vi "FGV Gaszuordnung Gas-Auswahl.vi"(6 "Aktion":T4, 8 "Graphen":T1, 10 "Auswahlfelder":T2, 11 "aktiver Graph":i32) -> (0 "Graphen":T1, 2 "Auswahlfelder OUT":T2, 3 "aktiver Graph":i32)   [LabVIEW 2020, in "Gaszuordnung AO.lvlib"]
uses:
  Gaszuordnung AO.lvlib
  Auswahlfelder Anzeige.ctl
  Visualisierungs Elemente/Auswahlfeld.ctl
  FGV Gaszuordnung Gas-Auswahl Aktion.ctl
  Grafik/Graphen Auswahl.ctl
  Allgemein/allgemeine Sub-VIs.lvlib
  Grafik/Grafik.lvlib
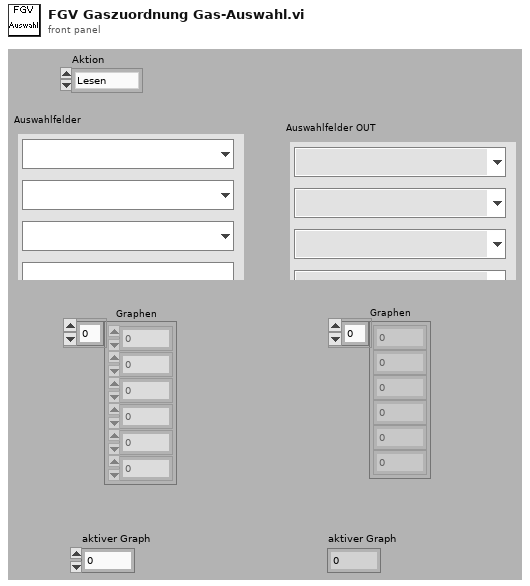
[diagram p1: front panel]
types:
  T1 = typedef "Grafik.lvlib/Graphen Auswahl.ctl" = u16[]
  T2 = typedef "Gaszuordnung AO.lvlib/Auswahlfelder Anzeige.ctl" = cluster{"Auswahl":T3, "Auswahl 2":T3, "Auswahl 3":T3, "Auswahl 4":T3, "Auswahl 5":T3, "Auswahl 6":T3, "Auswahl 7":T3, "Auswahl 8":T3, "Auswahl 9":T3, "Auswahl 10":T3, "Auswahl 11":T3, "Auswahl 12":T3, "Auswahl 13":T3, "Auswahl 14":T3, "Auswahl 15":T3, "Auswahl 16":T3}
  T3 = typedef "Auswahlfeld.ctl" = u16
  T4 = typedef "Gaszuordnung AO.lvlib/FGV Gaszuordnung Gas-Auswahl Aktion.ctl" = enum16{"Lesen", "AO Auswahl", "Graph Auswahl", "aktiver Graph", "laden", "speichern"}
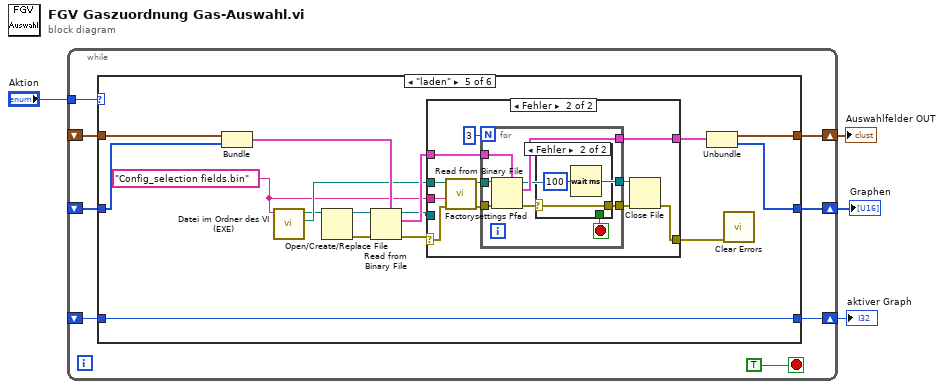
[diagram p0: block diagram]
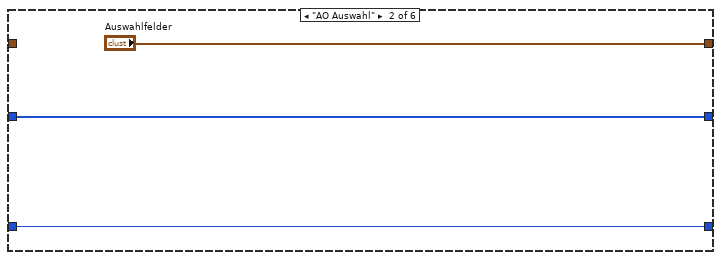
[diagram p3: hidden frame]
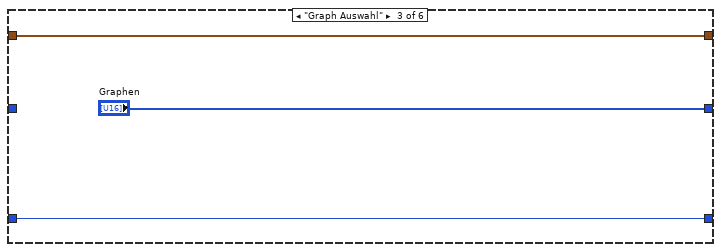
[diagram p4: hidden frame]
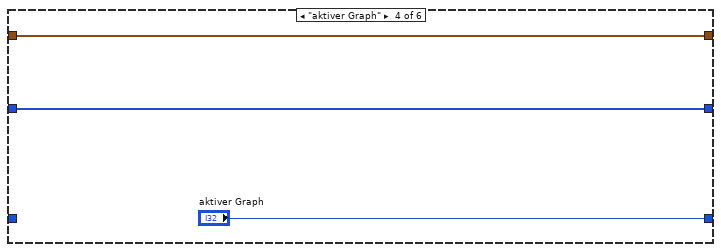
[diagram p5: hidden frame]
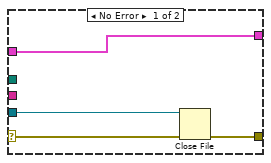
[diagram p6: hidden frame]
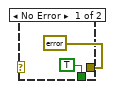
[diagram p7: hidden frame]
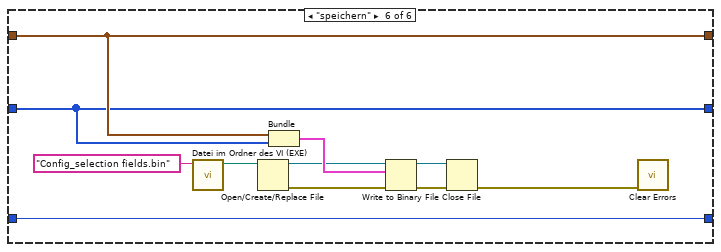
[diagram p8: hidden frame]
diagram:
  n1 = while {
    tunnel: "Aktion" -> [w11]
    shift-right: [w10] -> w3
    shift-left: _ -> [w9]
    shift-right: [w8] -> w2
    shift-left: _ -> [w7]
    shift-right: [w6] -> w1
    shift-left: _ -> [w5]
    stop <- TRUE stop-if-true
    n2 = case shown="\"laden\"" w11 {
      tunnel: [w15 "Auswahlfelder" w20 w22 w37 w77] -> w10
      tunnel: w9 -> [w15 _ w20 w22 w40 w77]
      tunnel: [w14 w17 "Graphen" w23 w36 w76] -> w8
      tunnel: w7 -> [w14 w17 _ w23 w39 w76]
      tunnel: [w13 w16 w19 "aktiver Graph" w35 w74] -> w6
      tunnel: w5 -> [w13 w16 w19 _ w35 w74]
      frame "Lesen", Default {
      }
      frame "AO Auswahl" {
      }
      frame "Graph Auswahl" {
      }
      frame "aktiver Graph" {
      }
      frame "laden" {
        w28 = "Config_selection fields.bin" ("Dateiname")
        n3 = Bundle("Auswahlfelder"=w40, "Graphen"=w39) -> (w38:cluster{"Auswahlfelder":T2, "Graphen":T1})  [unwired: 1 in]
        n4 = call "Datei im Ordner des VI (EXE).vi"("Dateiname"=w28) -> ("Ordner des Haupt-VIs"=w32:path, "Dateipfad im Ordner des Haupt-VIs"=w27:path)  [unwired: 8 in, 1 out]
        n5 = Open/Create/Replace File(file path (use dialog)=w27) -> (refnum out=w26:refnum<file>, error out=w25:errorcluster)  [unwired: 5 in, 1 out]
        n6 = Read from Binary File(5:w38, 8:w25, 11:w26) -> (0:w34:errorcluster, 2:w33:cluster{"Auswahlfelder":T2, "Graphen":T1}, 3:w31:refnum<file>)  [unwired: 3 in, 1 out]
        n7 = case shown="Fehler" w34 {
          selector: w34 -> [w43 w47]
          tunnel: w32 -> [_ w48]
          tunnel: w33 -> [w44 w46]
          tunnel: [w44 w54] -> w29
          tunnel: [w41 w52] -> w30
          tunnel: w31 -> [w42 _]
          tunnel: w28 -> [_ w45]
          frame No Error {
            n8 = Close File(refnum=w42, error in=w43) -> (error out=w41:errorcluster)  [unwired: 1 out]
          }
          frame Error {
            n9 = call "Factorysettings Pfad.vi"("error in (no error)"=w47, "Dateiname"=w45, "Ordner des Haupt-VIs"=w48) -> ("error out"=w49:errorcluster, "Pfad Factorysettings"=w50:path)  [unwired: 7 in]
            n10 = for {
              N: 3 -> [_]
              tunnel: w49 -> [w61]
              tunnel: w50 -> [w60]
              tunnel: [w59] -> w54
              tunnel: [w58] -> w53
              tunnel: [w57] -> w51
              tunnel: w46 -> [w56]
              stop <- w62 stop-if-true
              n11 = Read from Binary File(5:w56, 8:w61, 11:w60) -> (0:w63:errorcluster, 2:w59:cluster{"Auswahlfelder":T2, "Graphen":T1}, 3:w57:refnum<file>)  [unwired: 3 in, 1 out]
              n12 = case shown="Fehler" w63 {
                selector: w63 -> [_ w66]
                tunnel: [TRUE _] -> w62
                tunnel: [errorcluster {"status"=FALSE, "code"=0, "source"=""} ("error IO") w66] -> w58
                frame No Error {
                }
                frame Error {
                  n13 = Wait (ms)(milliseconds to wait=u32 100 ("Zu wartende ms")) -> ()  [unwired: 1 out]
                }
              }
            }
            n14 = Close File(refnum=w51, error in=w53) -> (error out=w52:errorcluster)  [unwired: 1 out]
          }
        }
        n15 = Unbundle(w29) -> ("Auswahlfelder"=w37:T2, "Graphen"=w36:T1)
        n16 = call <vilib>:"Clear Errors.vi"("error in (no error)"=w30) -> ()  [unwired: 5 in, 2 out]
      }
      frame "speichern" {
        n17 = call "Datei im Ordner des VI (EXE).vi"("Dateiname"="Config_selection fields.bin") -> ("Dateipfad im Ordner des Haupt-VIs"=w73:path)  [unwired: 8 in, 2 out]
        n18 = Open/Create/Replace File(file path (use dialog)=w73) -> (refnum out=w72:refnum<file>, error out=w71:errorcluster)  [unwired: 5 in, 1 out]
        n19 = Bundle("Auswahlfelder"=w77, "Graphen"=w76) -> (w75:cluster{"Auswahlfelder":T2, "Graphen":T1})  [unwired: 1 in]
        n20 = Write to Binary File(file (use dialog)=w72, data=w75, error in=w71) -> (refnum out=w68:refnum<file>, error out=w70:errorcluster)  [unwired: 3 in, 1 out]
        n21 = Close File(refnum=w68, error in=w70) -> (error out=w69:errorcluster)  [unwired: 1 out]
        n22 = call <vilib>:"Clear Errors.vi"("error in (no error)"=w69) -> ()  [unwired: 5 in, 2 out]
      }
    }
  }
  "Auswahlfelder OUT" <- w3
  "Graphen" <- w2
  "aktiver Graph" <- w1
